vi "SubTelemetry.vi"(8 "error in (no error)":errorcluster, 11 "SALCommunicatorView in":refnum<class "SALCommunicatorView.lvclass">) -> (0 "error out":errorcluster, 3 "SALCommunicatorView out":refnum<class "SALCommunicatorView.lvclass">)   [LabVIEW 2016, in "SALCommunicatorView.lvclass"]
uses:
  SALCommunicatorView.lvclass
  ts_sallv_exa/SALLV_EXA.lvlib
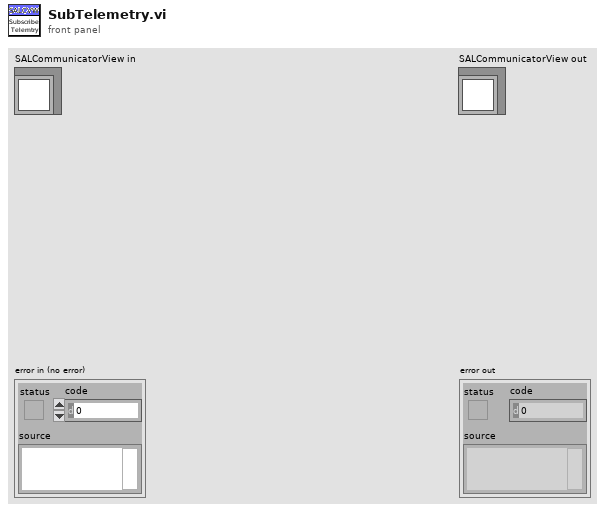
[diagram p1: front panel]
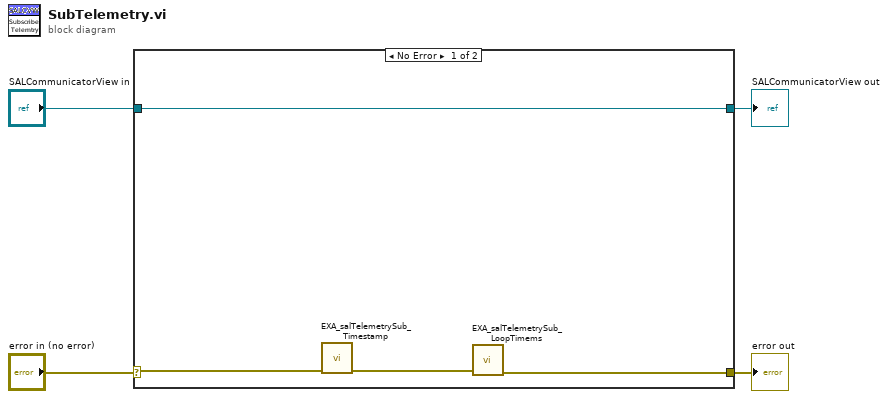
[diagram p0: block diagram]
diagram:
  n1 = case shown="No Error" "error in (no error)" {
    selector: "error in (no error)" -> [w5 w10]
    tunnel: [w7 w10] -> w3
    tunnel: [w8 w9] -> w1
    tunnel: "SALCommunicatorView in" -> [w8 w9]
    frame No Error {
      n2 = call "EXA_salTelemetrySub_Timestamp.vi"("error in (no error)"=w5) -> ("error out"=w6:errorcluster)  [unwired: 9 in, 1 out]
      n3 = call "EXA_salTelemetrySub_LoopTimems.vi"("error in (no error)"=w6) -> ("error out"=w7:errorcluster)  [unwired: 9 in, 1 out]
    }
    frame Error {
    }
  }
  "error out" <- w3
  "SALCommunicatorView out" <- w1
